vi "NextState_OA.vi"(6 "Ref?":bool, 8 "error in (no error)":errorcluster, 10 "Prop":T1={"Start/End"=enum."Start", "data"=[], "OrderAnalysis"={"dB on"=TRUE, "window type"=1, "max order to analyze"=32.0, "order resolution"=0.1, "Axis"=0, "Sample rate"=5000, "Save?"=FALSE, "Multiple_Frequency"=3, "averaging mode"=enum."No averaging"}, "Tacho"=[]} {"OrderAnalysis"."Axis" items=["X", "Y", "Z"]; "OrderAnalysis"."window type" items=["No averaging", "Vector averaging", "RMS averaging", "Peak hold"]}, 11 "Previous Step":T5) -> (0 "error out":errorcluster, 3 "Next Step":T5)   [LabVIEW 2021]
uses:
  Typedefs/State_OA.ctl
  Typedefs/PropertiesOrderAnalysis.ctl
  Typedefs/Start_End.ctl
  Typedefs/OrderAnalysis.ctl
  Typedefs/Axis.ctl
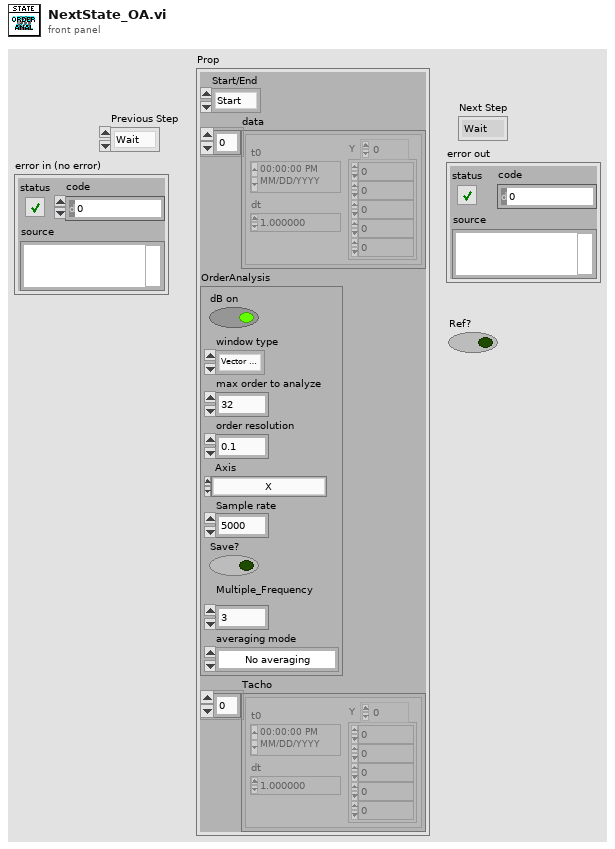
[diagram p1: front panel]
types:
  T1 = typedef "PropertiesOrderAnalysis.ctl" = cluster{"Start/End":T2, "data":waveform(dbl)[], "OrderAnalysis":T3, "Tacho":waveform(dbl)[]}
  T2 = typedef "Start_End.ctl" = enum16{"Start", "End"}
  T3 = typedef "OrderAnalysis.ctl" = cluster{"dB on":bool, "window type":u32, "max order to analyze":dbl, "order resolution":dbl, "Axis":T4, "Sample rate":i64, "Save?":bool, "Multiple_Frequency":i32, "averaging mode":enum16{"No averaging", "Vector averaging", "RMS averaging", "Peak hold"}}
  T4 = typedef "Axis.ctl" = u16
  T5 = typedef "State_OA.ctl" = enum16{"Wait", "Init", "Show", "Save"}
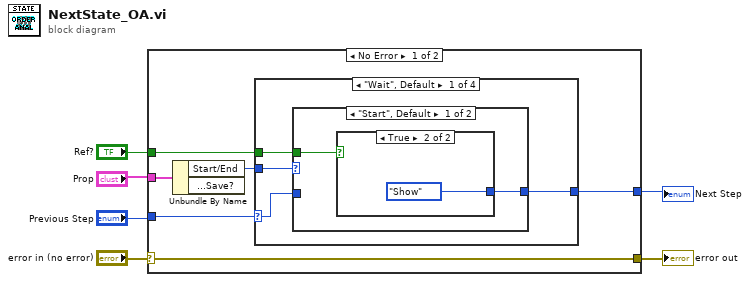
[diagram p0: block diagram]
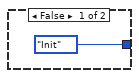
[diagram p2: hidden frame]
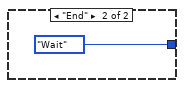
[diagram p3: hidden frame]
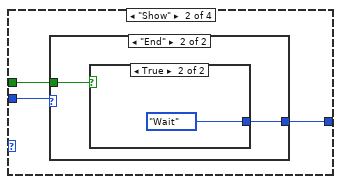
[diagram p4: hidden frame]
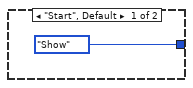
[diagram p5: hidden frame]
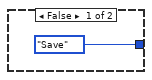
[diagram p6: hidden frame]
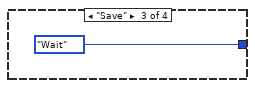
[diagram p7: hidden frame]
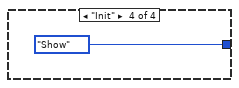
[diagram p8: hidden frame]
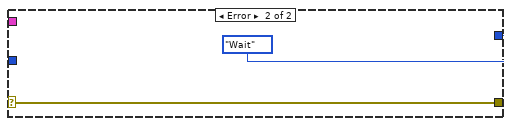
[diagram p9: hidden frame]
diagram:
  n1 = case shown="No Error" "error in (no error)" {
    selector: "error in (no error)" -> [w12 w33]
    tunnel: [w12 w33] -> w6
    tunnel: [w10 State_OA."Wait"] -> w3
    tunnel: "Prop" -> [w9 _]
    tunnel: "Previous Step" -> [w11 _]
    tunnel: "Ref?" -> [w7 _]
    frame No Error {
      n2 = Unbundle By Name(w9) -> ("Start/End"=w8:T2)  [unwired: 1 out]
      n3 = case shown="\"Wait\", Default" w11 {
        selector: w11 -> [w15 _ _ _]
        tunnel: w8 -> [w16 w24 _ _]
        tunnel: [w14 w23 State_OA."Wait" State_OA."Show"] -> w10
        tunnel: w7 -> [w13 w22 _ _]
        frame "Wait", Default {
          n4 = case shown="\"Start\", Default" w16 {
            tunnel: [w18 State_OA."Wait"] -> w14
            tunnel: w15 -> [_ _]
            tunnel: w13 -> [w17 _]
            frame "Start", Default {
              n5 = case shown="True" w17 {
                tunnel: [State_OA."Init" State_OA."Show"] -> w18
                frame False {
                }
                frame True {
                }
              }
            }
            frame "End" {
            }
          }
        }
        frame "Show" {
          n6 = case shown="\"End\"" w24 {
            tunnel: [State_OA."Show" w27] -> w23
            tunnel: w22 -> [_ w26]
            frame "Start", Default {
            }
            frame "End" {
              n7 = case shown="True" w26 {
                tunnel: [State_OA."Save" State_OA."Wait"] -> w27
                frame False {
                }
                frame True {
                }
              }
            }
          }
        }
        frame "Save" {
        }
        frame "Init" {
        }
      }
    }
    frame Error {
    }
  }
  "error out" <- w6
  "Next Step" <- w3
